vi "CAN_Start.vi"() -> (3 "Success":bool)   [LabVIEW 2020]
uses:
  Global_Variable/Global.vi
  Libraries/ZLG_CAN/ZLG_CAN.lvlib
panel:
  in  "CAN 通道":u32(ring) items=["0", "1"]
  in  "索引":u32(ring) items=["0", "1", "2", "3", "4", "5", "6", "7", "8"]
  in  "设备类型":u32(ring)=27 items=["PCI5121"=1, "PCI9810"=2, "USBCAN1"=3, "USBCAN2"=4, "PCI9820"=5, "PCI5110"=7, "PC104CAN"=11, "CANETUDP"=12, "PCI9840B"=14, "PC104C2"=15, "PCI9820I"=16, "CANETTCP"=17, "PCIE9221"=24, "PCI5010U"=19, "USBCAN_E_U"=20, "USBCAN_2E_U"=21, "PCI5020U"=22, "PCIE9120I"=27, "PCIE9110I"=28, "PCIE9140I"=29]
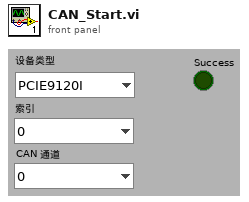
[diagram p1: front panel]
types:
  T1 = cluster{"波特率":u32, "ID":u32, "帧类型":enum8{"标准帧", "扩展帧"}, "帧格式":enum16{"数据帧", "远程帧"}, "周期(ms)":u32}
  T2 = typedef "ZLG_CAN.lvlib/Start_CAN (Reply Payload)--cluster.ctl" = cluster{"Success":bool, "Start_CAN_error":errorcluster}
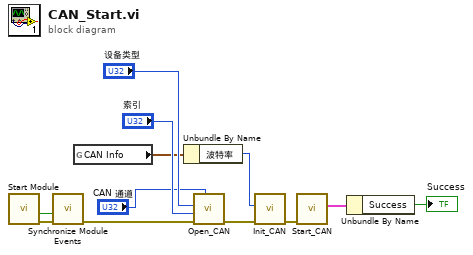
[diagram p0: block diagram]
diagram:
  n1 = call "Start Module.vi"() -> ("error out"=w12:errorcluster, "Wait for Event Sync?"=w11:bool)  [unwired: 8 in, 2 out]
  n2 = call "Synchronize Module Events.vi"("error in (no error)"=w12, "Wait for Event Sync?"=w11) -> ("error out"=w10:errorcluster)  [unwired: 9 in]
  n3 = global read "Global.vi" "CAN Info"() -> (w2:T1)
  n4 = Unbundle By Name(w2) -> ("波特率"=w3:u32)
  n5 = call "Open_CAN.vi"("CAN 通道"="CAN 通道", "error in (no error)"=w10, "索引"="索引", "设备类型"="设备类型") -> ("error out"=w7:errorcluster)  [unwired: 7 in]
  n6 = call "Init_CAN.vi"("error in (no error)"=w7, "波特率"=w3) -> ("error out"=w4:errorcluster)  [unwired: 9 in]
  n7 = call "Start_CAN.vi"("error in (no error)"=w4) -> ("Reply Payload"=w5:T2)  [unwired: 8 in, 2 out]
  n8 = Unbundle By Name(w5) -> ("Success"=→"Success":bool)
